vi "util_create_installer.vi"(8 "error in (no error)":errorcluster, 9 "archive":path, 10 "config":path, 11 "install_file in":path) -> (0 "error out":errorcluster, 3 "install_file out":path)   [LabVIEW 2015, in "lv-bin-7zip.lvlib"]
uses:
  lv-bin-7zip.lvlib
  <userlib>/antonio-alexander/lv-bin/lv-bin/public/api/v1/v1.lvlib
panel:
  out "standard_output":string
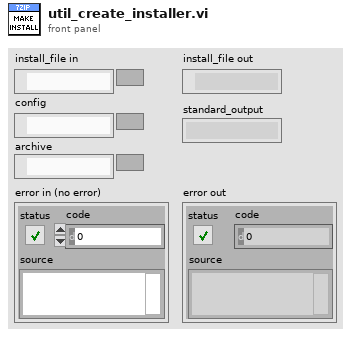
[diagram p1: front panel]
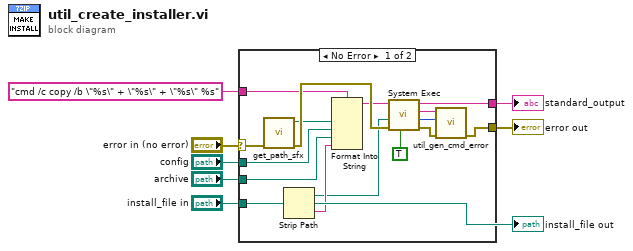
[diagram p0: block diagram]
diagram:
  n1 = case shown="No Error" "error in (no error)" {
    selector: "error in (no error)" -> [w9 w24]
    tunnel: "install_file in" -> [w22 _]
    tunnel: [w14 w24] -> w5
    tunnel: [w18 _] -> w1
    tunnel: "config" -> [w17 _]
    tunnel: "archive" -> [w16 _]
    tunnel: "cmd /c copy /b \"%s\" + \"%s\" + \"%s\" %s" ("format string") -> [w8 _]
    frame No Error {
      n2 = call "get_path_sfx.vi"("error in (no error)"=w9) -> ("error out"=w23:errorcluster, "sfx"=w11:path)  [unwired: 9 in]
      n3 = Strip Path(path=w22) -> (stripped path=w20:path, name=w21:string)
      n4 = Format Into String(format string=w8, w11, w17, w16, w21) -> (resulting string=w19:string)  [unwired: 2 in, 1 out]
      n5 = call <vilib>:"System Exec.vi"("run minimized? (F)"=TRUE, "error in (no error)"=w23, "working directory"=w20, "command line"=w19) -> ("error out"=w15:errorcluster, "return code"=w10:i32, "standard error"=w12:string, "standard output"=w18:string)  [unwired: 4 in]
      n6 = call <userlib>:"util_gen_cmd_error.vi"("error in (no error)"=w15, "return_code"=w10, "standard_error"=w12) -> ("error out"=w14:errorcluster)  [unwired: 8 in]
    }
    frame Error {
    }
  }
  "error out" <- w5
  "standard_output" <- w1
  "install_file out" <- "install_file in"
